vi "SUBVItest.vi"() -> ()   [LabVIEW 2017]
uses:
  <instrlib>/Keysight N8900 Series/Public/Data/Read Output (Voltage).vi
  <instrlib>/Keysight N8900 Series/Keysight N8900 Series.lvlib
panel:
  in  "VISA resource name":refnum<visa-resource-name>="TCPIP0::A-N8731A-8956R.local::inst0::INSTR"
  in  "Reset (True)":bool=TRUE
  out "read buffer":string
  in  "write buffer":string
  out "Constant Current Mode":bool
  out "Constant Voltage Mode":bool
  out "Voltage Level":dbl
  out "Instrument Firmware Revision":string
  out "Instrument Driver Revision":string
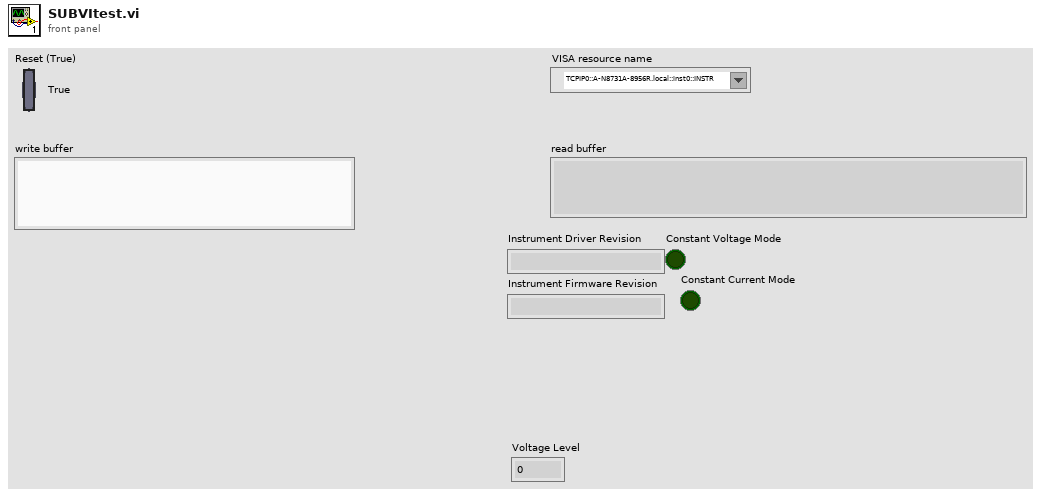
[diagram p1: front panel]
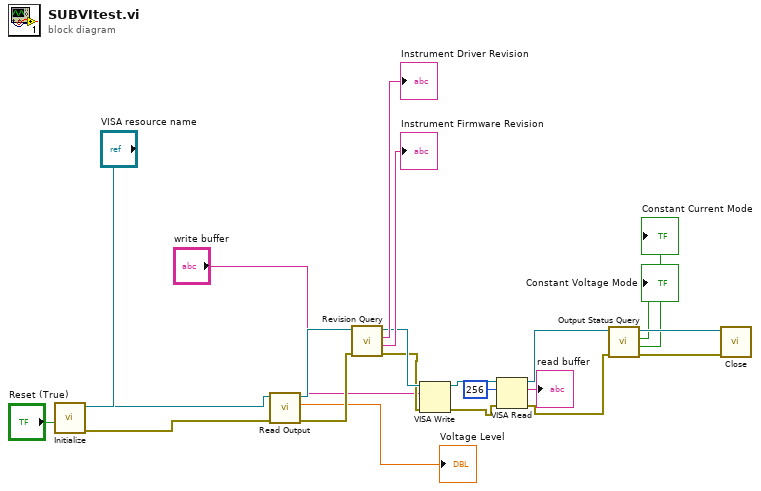
[diagram p0: block diagram]
diagram:
  n1 = call <instrlib>:"Initialize.vi"("Reset (True)"="Reset (True)", "VISA resource name"="VISA resource name") -> ("error out"=w4:errorcluster, "VISA resource name out"=w5:refnum<visa-resource-name>)  [unwired: 8 in]
  n2 = call-poly <instrlib>:"Read Output.vi"("error in (no error)"=w4, "VISA resource name"=w5) -> ("error out"=w19:errorcluster, "Voltage Level"=→"Voltage Level":dbl, "VISA resource name out"=w18:refnum<visa-resource-name>)  [unwired: 7 in]
  n3 = call <instrlib>:"Revision Query.vi"("error in (no error)"=w19, "VISA resource name"=w18) -> ("error out"=w11:errorcluster, "Instrument Firmware Revision"=→"Instrument Firmware Revision":string, "Instrument Driver Revision"=→"Instrument Driver Revision":string, "VISA resource name out"=w12:refnum<visa-resource-name>)  [unwired: 6 in]
  n4 = VISA Write(VISA resource name=w12, write buffer="write buffer", error in (no error)=w11) -> (VISA resource name out=w8:refnum<visa-resource-name>, error out=w9:errorcluster)  [unwired: 1 out]
  n5 = VISA Read(VISA resource name=w8, byte count=u32 256, error in (no error)=w9) -> (VISA resource name out=w2:refnum<visa-resource-name>, read buffer=→"read buffer":string, error out=w1:errorcluster)  [unwired: 1 out]
  n6 = call <instrlib>:"Output Status Query.vi"("error in (no error)"=w1, "VISA resource name"=w2) -> ("error out"=w16:errorcluster, "Constant Current Mode"=→"Constant Current Mode":bool, "Constant Voltage Mode"=→"Constant Voltage Mode":bool, "VISA resource name out"=w15:refnum<visa-resource-name>)  [unwired: 6 in]
  n7 = call <instrlib>:"Close.vi"("error in (no error)"=w16, "VISA resource name"=w15) -> ()  [unwired: 9 in, 1 out]
